vi "macro_MedianFilter_Execute.vi"   [LabVIEW 2019, in "Trajectory_Library.lvlib"]
uses:
  Trajectory_Library.lvlib
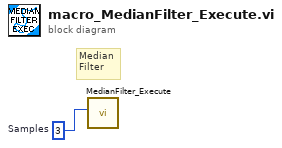
[diagram p0: block diagram]
diagram:
  w1 = 3  # Samples
  # "Median\nFilter"
  n1 = call "MedianFilter_Execute.vi"("Samples"=w1) -> ()  [unwired: 9 in, 2 out]
